vi "Launcher.vi"() -> ()   [LabVIEW 2021]
doc: "MIT Licence\nCopyright (c) 2024 David Grollier"
uses:
  Type Def/Game Settings.ctl
  Type Def/Control Device.ctl
  Type Def/Players Number.ctl
  Type Def/Difficulty.ctl
  Type Def/FPS.ctl
  Type Def/Mode.ctl
panel:
  in  "Game Settings":T1={"Control Device"=enum."Mouse", "Players Number"=2, "Score Limit"=3, "Difficulty"=0.8, "FPS"=8, "Mode"=enum."Solo"} {"FPS" items=["120"=8, "60"=16]; "Difficulty" items=["Hard"=1.0, "Medium"=0.8, "Easy"=0.6]; "Players Number" items=["2"=2, "4"=4]}
  in  "Quit":bool
  in  "Start":bool
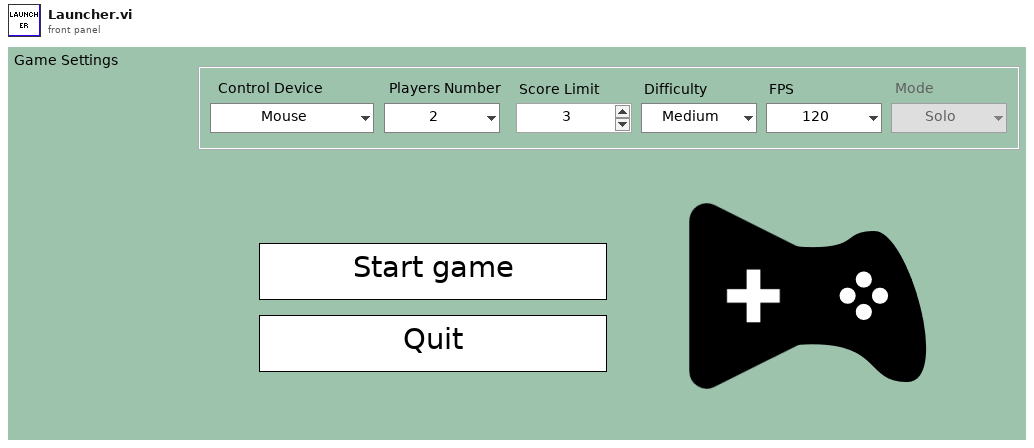
[diagram p1: front panel]
types:
  T1 = typedef "Game Settings.ctl" = cluster{"Control Device":T2, "Players Number":T3, "Score Limit":u8, "Difficulty":T4, "FPS":T5, "Mode":T6}
  T2 = typedef "Control Device.ctl" = enum16{"Arrow Keys", "Mouse", "Xbox Controller"}
  T3 = typedef "Players Number.ctl" = u16
  T4 = typedef "Difficulty.ctl" = dbl
  T5 = typedef "FPS.ctl" = u8
  T6 = typedef "Mode.ctl" = enum16{"Solo", "Multiplayer"}
  T7 = enum32{"Invalid", "Standard", "Closed", "Hidden", "Minimized", "Maximized"}
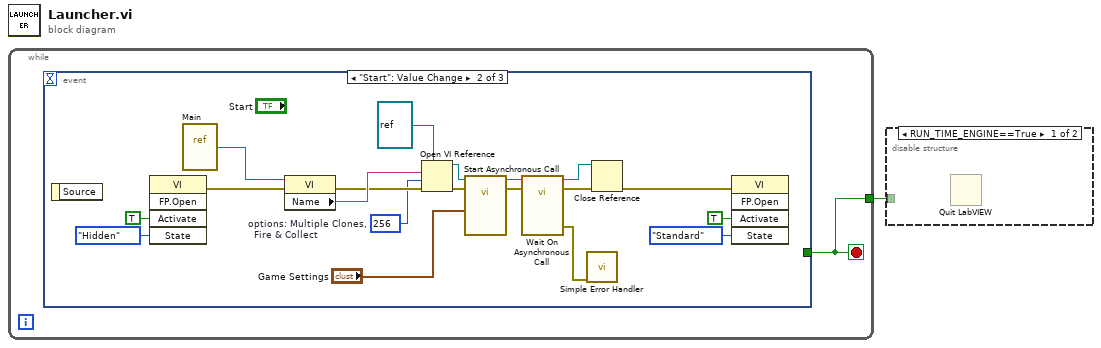
[diagram p0: block diagram]
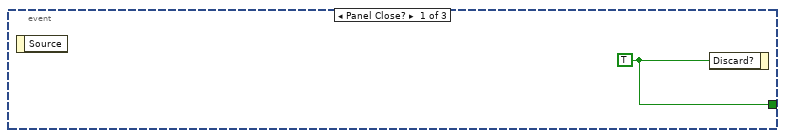
[diagram p3: hidden frame]
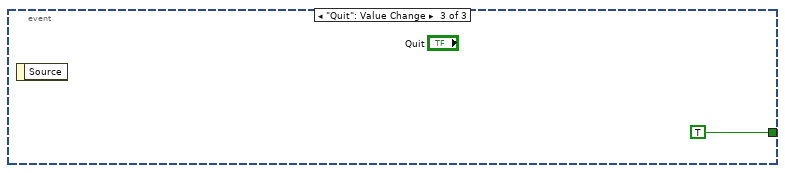
[diagram p4: hidden frame]
diagram:
  n1 = while {
    tunnel: [w2] -> w1
    stop <- w2 stop-if-true
    n2 = event shown="[1] \"Start\": Value Change" {
      selector: _ -> [_ _ _]
      dyn-events: _ -> [_ _ _]
      timeout: _ -> [_ _ _]
      tunnel: [w3 _ TRUE ("Discard?")] -> w2
      event Panel Close? {
        w3 = TRUE ("Discard?")
        n3 = event-data() -> ()  [unwired: 1 in, 1 out]
        n4 = event-data("Discard?"=w3) -> ()  [unwired: 1 in, 1 out]
      }
      event "Start": Value Change {
        w12 = 256  # options: Multiple Clones,   Fire & Collect
        n5 = event-data() -> ()  [unwired: 1 in, 1 out]
        n6 = invoke class="VI" method="FP.Open"("Activate"=TRUE ("Activate?"), "State"=T7."Hidden") -> (error out=w8:errorcluster)  [unwired: 3 in, 4 out]
        n7 = vi-ref "Main.vi"() -> (w16:refnum<vi>)
        n8 = property class="VI"(reference=w16, error in=w8) -> (error out=w14:errorcluster, "Name"=w15:string)  [unwired: 1 out]
        n9 = Open VI Reference(type specifier VI Refnum (for type only)=refnum<vi> refnum, vi path=w15, options=w12, error in (no error)=w14) -> (vi reference=w21:refnum<vi>, error out=w22:errorcluster)  [unwired: 2 in]
        n10 = call-by-ref "Start Asynchronous Call"(reference=w21, error in=w22, "Game Settings"="Game Settings") -> (reference out=w18:refnum<vi>, error out=w17:errorcluster)  [unwired: 10 in, 1 out]
        n11 = call-by-ref "Wait On Asynchronous Call"(reference=w18, error in=w17) -> (reference out=w20:refnum<vi>, error out=w19:errorcluster, 0:"error out"=w5:errorcluster)  [unwired: 11 in]
        n12 = call <vilib>:"Simple Error Handler.vi"("error in (no error)"=w5) -> ()  [unwired: 4 in, 5 out]
        n13 = Close Reference(reference=w20, error in (no error)=w19) -> (error out=w9:errorcluster)
        n14 = invoke class="VI" method="FP.Open"(error in=w9, "Activate"=TRUE ("Activate?"), "State"=T7."Standard") -> ()  [unwired: 2 in, 5 out]
      }
      event "Quit": Value Change {
        n15 = event-data() -> ()  [unwired: 1 in, 1 out]
      }
    }
  }
  n16 = disable-structure shown="RUN_TIME_ENGINE==True" {
    disable-tunnel: w1 -> [_ _]
    frame condition #0 {
      n17 = Quit LabVIEW() -> ()  [unwired: 1 in]
    }
    frame condition #1 (active) {
    }
  }
